vi "SUBVI_filesave_subVI-lm-mdk.vi"(4 "Height":dbl, 6 "Width":dbl, 8 "error in":errorcluster, 10 "Sample Name":string) -> (0 "error out":errorcluster, 2 "bin path":path, 3 "refnum out":refnum<file>)   [LabVIEW 2020]
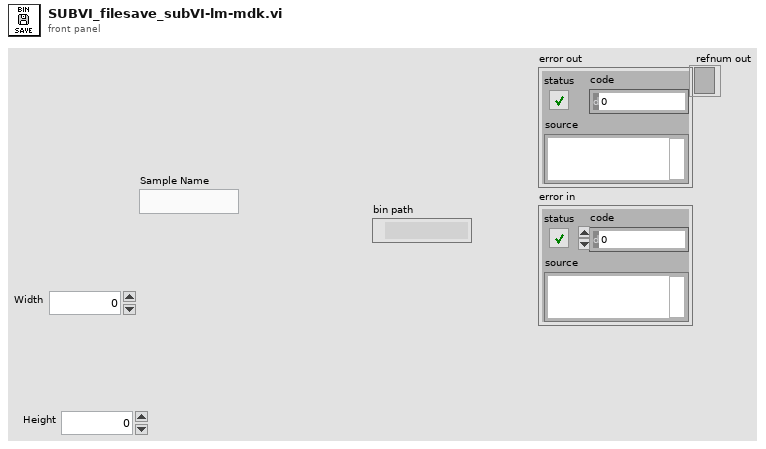
[diagram p1: front panel]
types:
  T1 = enum16{"open", "replace", "create", "open or create", "replace or create", "replace or create with confirmation"}
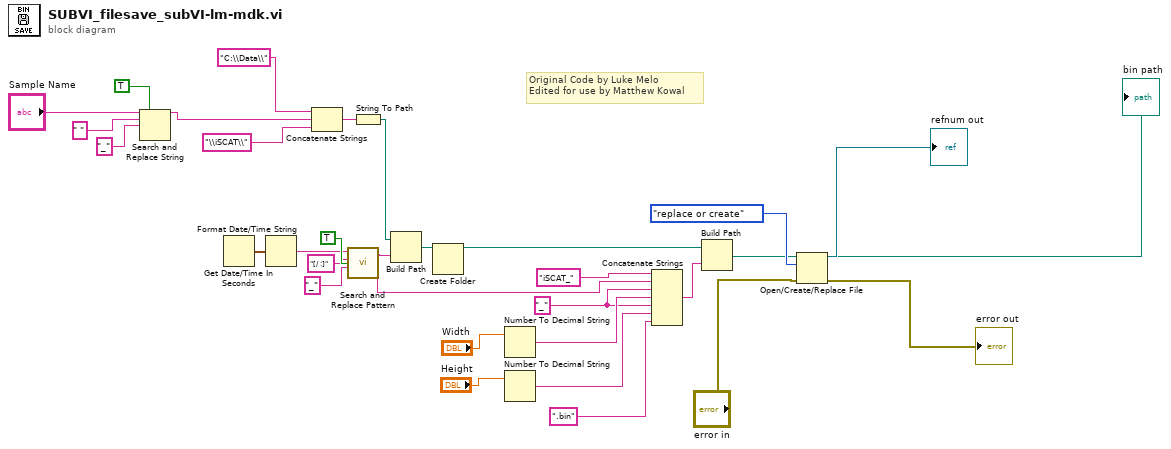
[diagram p0: block diagram]
diagram:
  w3 = "_"
  # "Original Code by Luke Melo\nEdited for use by Matthew Kowal"
  n1 = Search and Replace String(replace all?=TRUE ("replace all? (F)"), input string="Sample Name", search string=" ", replace string="_" ("replace string (\"\")")) -> (result string=w15:string)  [unwired: 4 in, 3 out]
  n2 = Get Date/Time In Seconds() -> (seconds since 1Jan1904=w26:timestamp)
  n3 = Format Date/Time String(seconds (now)=w26) -> (date/time string=w27:string)  [unwired: 2 out]
  n4 = Concatenate Strings("C:\\Data\\" ("string"), w15, "\\iSCAT\\" ("string")) -> (w14:string)
  n5 = call <vilib>:"Search and Replace Pattern.vi"("string"=w27, "regular expression (\"\")"="[/ :]", "replace string (\"\")"="_", "replace all? (F)"=TRUE) -> ("result string"=w21:string)  [unwired: 1 in, 1 out]
  n6 = String To Path(string=w14) -> (path=w8:path)
  n7 = Build Path(base path=w8, name or relative path=w21) -> (appended path=w25:path)
  n8 = Create Folder(path (use dialog)=w25) -> (created path=w24:path)  [unwired: 2 in, 2 out]
  n9 = Number To Decimal String(number="Width") -> (decimal integer string=w4:string)  [unwired: 1 in]
  n10 = Number To Decimal String(number="Height") -> (decimal integer string=w2:string)  [unwired: 1 in]
  n11 = Concatenate Strings("iSCAT_", w21, w3, w4, w3, w2, ".bin") -> (w23:string)
  n12 = Build Path(base path=w24, name or relative path=w23) -> (appended path=w16:path)
  "bin path" <- w16
  n13 = Open/Create/Replace File(file path (use dialog)=w16, error in="error in", operation (0:open)=T1."replace or create") -> (refnum out=→"refnum out":refnum<file>, error out=→"error out":errorcluster)  [unwired: 3 in, 1 out]
